vi "instance count allowed.vi"(8 "error in":errorcluster, 11 "Daqmx Module configuration in":refnum<class "DAQmx Module Configuration.lvclass">) -> (0 "error out":errorcluster, 2 "instances allowed":i32, 3 "Daqmx Module configuration out":refnum<class "DAQmx Module Configuration.lvclass">)   [LabVIEW 2014, in "DAQmx Module Configuration.lvclass"]
uses:
  DAQmx Module Configuration.lvclass
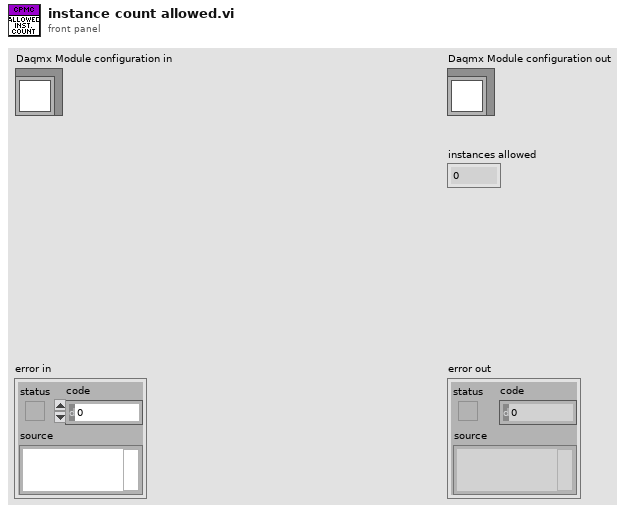
[diagram p1: front panel]
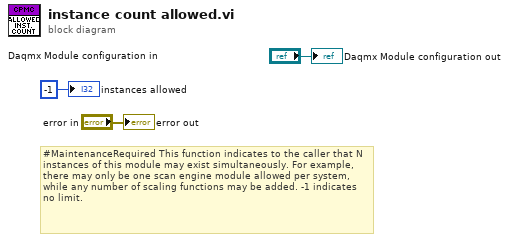
[diagram p0: block diagram]
diagram:
  # "#MaintenanceRequired This function indicates to the caller that N instances of this module may exist simultaneously. For example, there may only be one scan engine module allowed per system, while any number of scaling functions may be added. -1 indicates no limit."
  "error out" <- "error in"
  "Daqmx Module configuration out" <- "Daqmx Module configuration in"
  "instances allowed" <- -1 ("instances allowed")
